vi "Update FF.vi"(4 "b0":fxp<+/-,32,2>, 5 "Reset":bool=TRUE, 6 "a0":fxp<+/-,32,2>, 7 "source adress":u32, 8 "input valid":bool=TRUE, 9 "destination adress":u32, 10 "Destination memory":refnum<k21>="Beam_I", 11 "Source memory":refnum<k21>="Adaptive FF I") -> (0 "output valid":bool)   [LabVIEW 2018]
uses:
  <vilib>/rvi/DataTransferAndStorage/Container/Common/niFpgaContainerExecOnDevCompGetState.vi
  <vilib>/rvi/Emulation/niFpgaEmulationIsFPGAContextNoSignature.vi
  <vilib>/rvi/DataTransferAndStorage/Container/Common/niFpgaContainerGetUniqueNameForEmu.vi
  <vilib>/rvi/Emulation/niFpgaProcessEmulError.vi
  <vilib>/rvi/Emulation/niFpgaSctlEmulationGetInTimedLoop.vi
  <vilib>/rvi/errors/nirviReportUnexpectedCaseInternalError (U32).vi
  <vilib>/rvi/Memory/Memory_Emulation/niFpgaMemoryEmulationCacheClearOnFirstRun.vi
  <vilib>/rvi/Memory/Memory_Emulation/nirvimemoryEmulationManagerCache_MakeExclusive.vi
  <vilib>/rvi/Memory/Memory_Emulation/niFpgaMemoryEmulationValidateCache.vi
  <vilib>/rvi/Memory/Memory_Emulation/nirvimemoryEmulationManagerCache_InsertValue.vi
  <vilib>/Utility/error.llb/Clear Errors.vi
  <vilib>/rvi/Memory/Memory_Emulation/nirvimemoryEmulationManagerCache_ReleaseExclusive.vi
  <vilib>/rvi/Memory/Memory_Emulation/nirvimemoryEmulationManagerCache_GetValue.vi
  <vilib>/rvi/Memory/Memory_Emulation/nirvimemoryEmulationManagerCache_SetValue.vi
  <vilib>/rvi/Emulation/niFpgaSctlEmulationResourceMgr.vi
  <vilib>/rvi/DataTransferAndStorage/Container/XNode/niFpgaContainer.xnode
  <vilib>/rvi/Memory/Memory_Emulation/niFpgaMemoryEmulationRefIn.vi
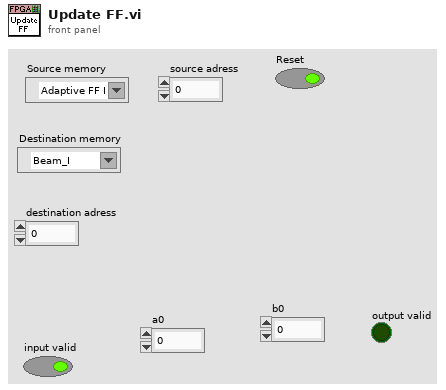
[diagram p1: front panel]
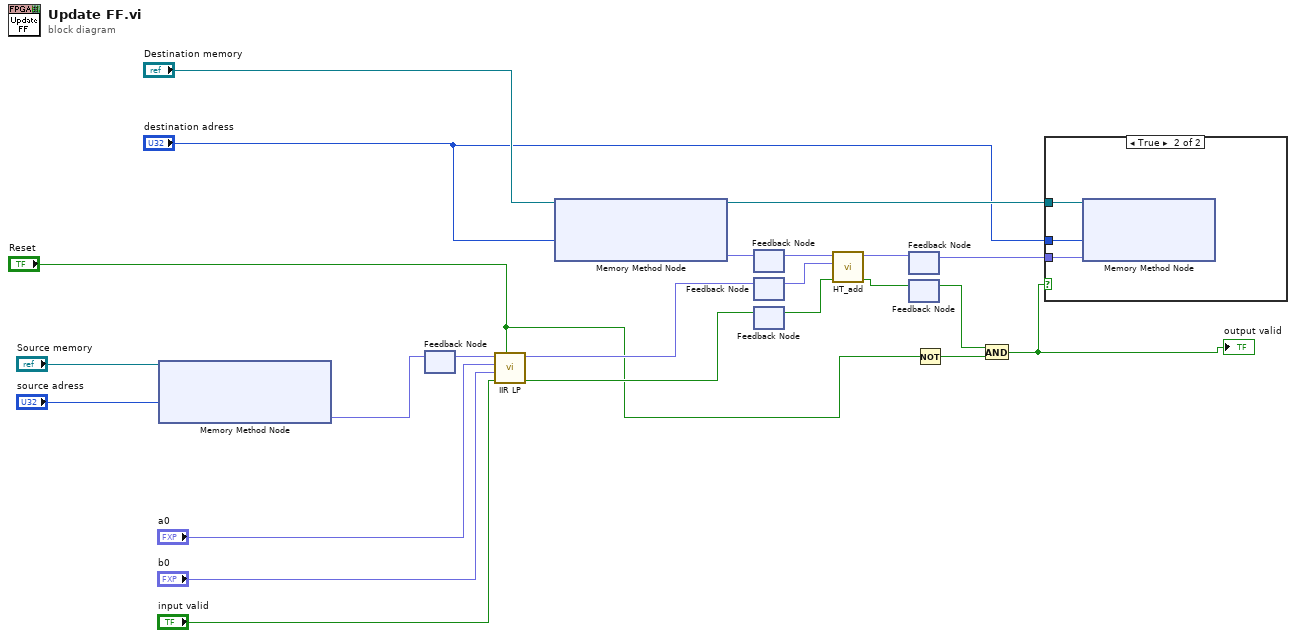
[diagram p0: block diagram]
diagram:
  n1 = xnode ("Memory Method Node")("Address"="source adress", "Memory In"="Source memory") -> ("Data"=w21:fxp<+/-,16,14>)  [unwired: 1 out]
  n2 = feedback-in #1(w21) -> ()
  n3 = feedback #1() -> (w20:fxp<+/-,16,14>)  [unwired: 1 in]
  n4 = call "IIR LP.vi"("Reset"="Reset", "input valid"="input valid", "b0"="b0", "a0"="a0", "Value in"=w20) -> ("output valid"=w9:bool, "Value out"=w10:fxp<+/-,16,14>)  [unwired: 5 in]
  n5 = xnode ("Memory Method Node")("Address"="destination adress", "Memory In"="Destination memory") -> ("Data"=w11:fxp<+/-,16,14>, "Memory Out"=w16:refnum<k21>)
  n6 = feedback #2() -> (w12:fxp<+/-,16,14>)  [unwired: 1 in]
  n7 = feedback-in #2(w11) -> ()
  n8 = feedback #3() -> (w13:fxp<+/-,16,14>)  [unwired: 1 in]
  n9 = feedback-in #3(w10) -> ()
  n10 = feedback #4() -> (w14:bool)  [unwired: 1 in]
  n11 = feedback-in #4(w9) -> ()
  n12 = call "HT_add.vi"("input valid"=w14, "y"=w13, "x"=w12) -> ("output valid"=w6:bool, "x+y"=w8:fxp<+/-,16,14>)  [unwired: 7 in]
  n13 = feedback #5() -> (w7:fxp<+/-,16,14>)  [unwired: 1 in]
  n14 = feedback-in #5(w8) -> ()
  n15 = feedback #6() -> (w3:bool)  [unwired: 1 in]
  n16 = feedback-in #6(w6) -> ()
  n17 = Not(x="Reset") -> (.not. x?=w4:bool)
  n18 = And(x=w3, y=w4) -> (x .and. y?=w1:bool)
  "output valid" <- w1
  n19 = case shown="True" w1 {
    tunnel: w16 -> [_ w26]
    tunnel: w7 -> [_ w25]
    tunnel: "destination adress" -> [_ w24]
    frame False {
    }
    frame True {
      n20 = xnode ("Memory Method Node")("Address"=w24, "Data"=w25, "Memory In"=w26) -> ()  [unwired: 1 out]
    }
  }
